vi "add set temp(SubVI).vi"(6 "limit":T1, 10 "字符串":string) -> (0 "布尔 3":bool, 2 "连接的字符串":string)   [LabVIEW 2019, in "Add Seq.lvlib"]
uses:
  Add Seq.lvlib
  ctl/limit.ctl
  SubVI.lvlib
panel:
  in  "Mode":i32(ring) items=["FastSettle", "NoOvershoot"]
  in  "cancel":bool
  in  "ok":bool
  in  "Rate(K/min)":dbl=10.0 min=0.0 max=10.0
  in  "Temperature(K)":dbl=2.0 min=2.0 max=325.0
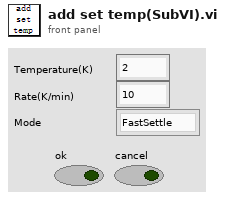
[diagram p1: front panel]
types:
  T1 = typedef "limit.ctl" = cluster{"Field limit":dbl, "Field rate limit":dbl, "Temp limit":dbl, "Temp low limit":dbl, "Temp rate limit ":dbl}
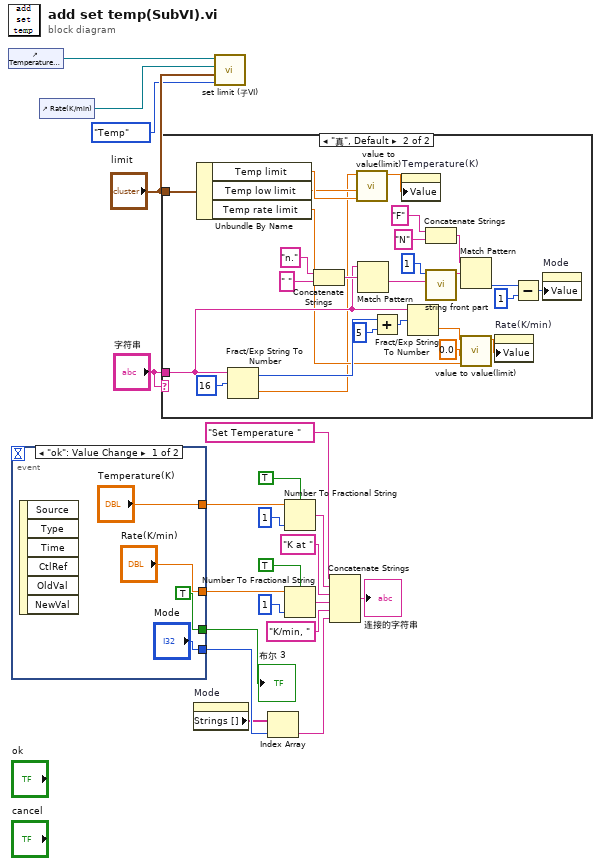
[diagram p0: block diagram]
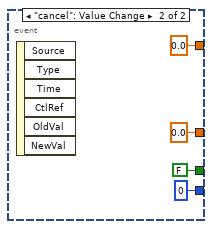
[diagram p3: hidden frame]
diagram:
  n1 = control-ref of="Temperature(K)"() -> (w4:refnum<vi>)
  n2 = event shown="[0] \"ok\": Value Change" {
    selector: _ -> [_ _]
    dyn-events: _ -> [_ _]
    timeout: _ -> [_ _]
    tunnel: ["Rate(K/min)" 0.0 ("Rate输入")] -> w12
    tunnel: ["Temperature(K)" 0.0 ("Field")] -> w19
    tunnel: [TRUE FALSE] -> w21
    tunnel: ["Mode" 0 ("Approach输入")] -> w9
    event "ok": Value Change {
      n3 = event-data() -> ()  [unwired: 1 in, 6 out]
    }
    event "cancel": Value Change {
      n4 = event-data() -> ()  [unwired: 1 in, 6 out]
    }
  }
  "布尔 3" <- w21
  n5 = control-ref of="Rate(K/min)"() -> (w3:refnum<vi>)
  n6 = case shown="\"真\", Default" "字符串" {
    tunnel: "字符串" -> [_ w39]
    tunnel: "limit" -> [_ w38]
    frame "" {
    }
    frame "真", Default {
      n7 = Unbundle By Name(w38) -> ("Temp limit"=w37:dbl, "Temp low limit"=w36:dbl, "Temp rate limit"=w35:dbl)
      n8 = Fract/Exp String To Number(string=w39, offset=16 ("偏移量")) -> (offset past number=w54:i32, number=w31:dbl)  [unwired: 2 in]
      n9 = Concatenate Strings("n." ("正则表达式"), " " ("字符串")) -> (w41:string)
      n10 = call "value to value(limit).vi"("high limit"=w37, "low limit"=w36, "数值 in"=w31) -> ("数值 out"=w30:dbl)  [unwired: 8 in]
      n11 = Match Pattern(string=w39, regular expression=w41) -> (after substring=w44:string)  [unwired: 1 in, 3 out]
      n12 = Add(x=w54, y=5) -> (x+y=w53:i32)
      n13 = property on="Temperature(K)" class="DigNum (strict)"("Value"=w30) -> ()  [unwired: 2 in, 2 out]
      n14 = Fract/Exp String To Number(string=w39, offset=w53) -> (number=w33:dbl)  [unwired: 2 in, 1 out]
      n15 = Concatenate Strings("F" ("字符串"), "N" ("字符串")) -> (w47:string)
      n16 = call "string front part.vi"("字符串"=w44, "偏移量(0)"=1) -> ("result string"=w50:string)  [unwired: 9 in]
      n17 = Match Pattern(string=w47, regular expression=w50) -> (offset past match=w46:i32)  [unwired: 1 in, 3 out]
      n18 = call "value to value(limit).vi"("high limit"=w35, "low limit"=0.0, "数值 in"=w33) -> ("数值 out"=w32:dbl)  [unwired: 8 in]
      n19 = property on="Rate(K/min)" class="DigNum (strict)"("Value"=w32) -> ()  [unwired: 2 in, 2 out]
      n20 = Subtract(x=w46, y=1) -> (x-y=w40:i32)
      n21 = property on="Mode" class="Ring (strict)"("Value"=w40) -> ()  [unwired: 2 in, 2 out]
    }
  }
  n22 = property on="Mode" class="Ring (strict)"() -> ("Strings []"=w6:string[])  [unwired: 2 in, 2 out]
  n23 = call "set limit (子VI).vi"("Temp or Field"=enum16{"Field", "Temp"}."Temp", "limit"="limit", "rate"=w3, "value"=w4) -> ()  [unwired: 8 in]
  n24 = Index Array(array=w6, index=w9) -> (element=w8:string)
  n25 = Number To Fractional String(use system decimal point (T)=TRUE ("使用系统小数点(T)"), number=w19, precision (6)=i16 1 ("精度(6)")) -> (F-format string=w17:string)  [unwired: 1 in]
  n26 = Number To Fractional String(use system decimal point (T)=TRUE ("使用系统小数点(T)"), number=w12, precision (6)=i16 1 ("精度(6)")) -> (F-format string=w11:string)  [unwired: 1 in]
  n27 = Concatenate Strings("Set Temperature " ("字符串"), w17, "K at " ("字符串"), w11, "K/min, " ("字符串"), w8) -> (→"连接的字符串":string)
